vi "Measure.vi"(8 "error in (no error)":errorcluster, 11 "VISA resource name":refnum<visa-resource-name>) -> (0 "error out":errorcluster, 2 "Output":string, 3 "VISA resource name out":refnum<visa-resource-name>)   [LabVIEW 2018, in "Keithley 3706.lvlib"]
uses:
  <instrlib>/Keithley 3706/Keithley 3706.lvlib
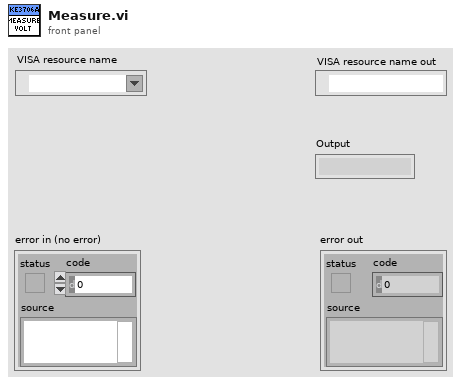
[diagram p1: front panel]
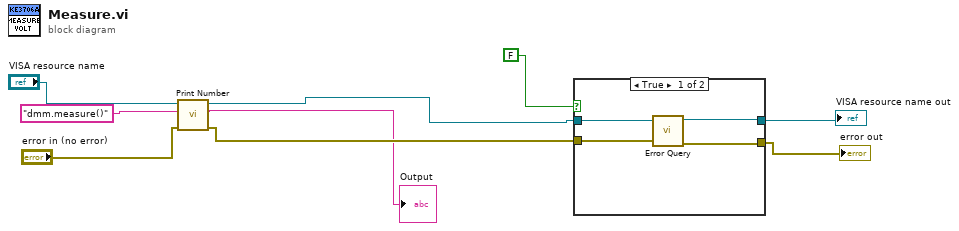
[diagram p0: block diagram]
diagram:
  n1 = call <instrlib>:"Print Number.vi"("error in (no error)"="error in (no error)", "Input"="dmm.measure()", "VISA resource name"="VISA resource name") -> ("error out"=w3:errorcluster, "Output"=→"Output":string, "VISA resource name out"=w1:refnum<visa-resource-name>)  [unwired: 5 in, 1 out]
  n2 = case shown="True" FALSE {
    tunnel: w1 -> [w13 w15]
    tunnel: w3 -> [w12 w14]
    tunnel: [w11 w15] -> w8
    tunnel: [w10 w14] -> w7
    frame True {
      n3 = call <instrlib>:"Error Query.vi"("error in (no error)"=w12, "VISA resource name"=w13) -> ("error out"=w10:errorcluster, "VISA resource name output"=w11:refnum<visa-resource-name>)  [unwired: 6 in, 2 out]
    }
    frame False {
    }
  }
  "VISA resource name out" <- w8
  "error out" <- w7
